vi "Status Tree to JSON.vi"(4 "Status Tree":map{string[], T1}(c390)) -> (7 "JSON":string)   [LabVIEW 2023, in "Volatus.lvlib" / "DebugHTTPController.lvclass"]
uses:
  DebugHTTPController.lvclass
  Module Status.ctl
  Module/State.ctl
  lv-cdm/CDM-Config/Config-JSON/Config-JSON.lvclass
  lv-cdm/CDM-Config/Config Element/Write Variant Value.vi
  DebugHTTPController.lvclass/DebugHTTPController.ctl
  lv-cdm/CDM-Config/Config Manager/Config Manager.lvclass
  lv-cdm/CDM-Config/Config Element/Config Element.lvclass
  Module/Module.lvclass
  Volatus.lvlib
panel:
  out "error out":errorcluster
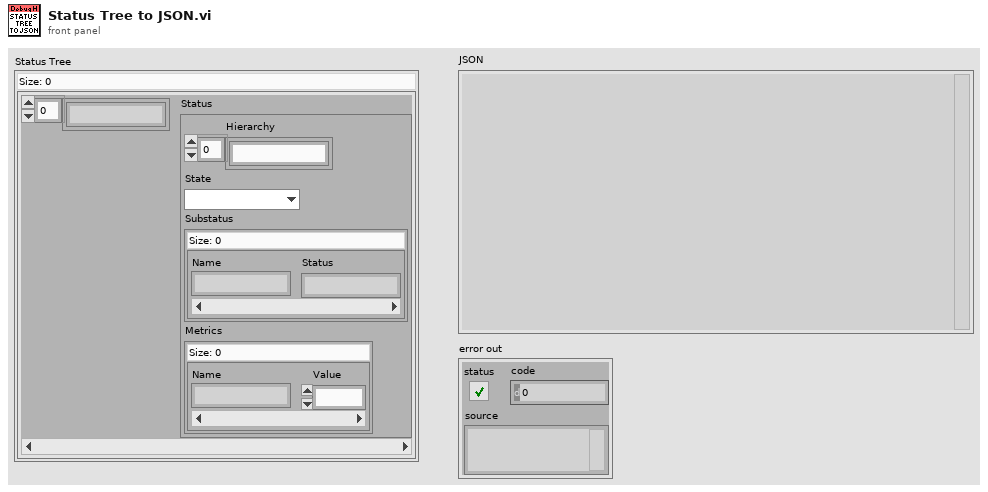
[diagram p1: front panel]
types:
  T1 = typedef "Volatus.lvlib/Module Status.ctl" = cluster{"Hierarchy":string[], "State":T2, "Substatus":map{string, string}, "Metrics":map{string, dbl}}
  T2 = typedef "Volatus.lvlib/Module.lvclass/State.ctl" = enum16{"Unknown", "Launched", "Starting", "Running", "Stopping", "Stopped", "Error - Starting", "Error - Run", "Error - Stopping"}
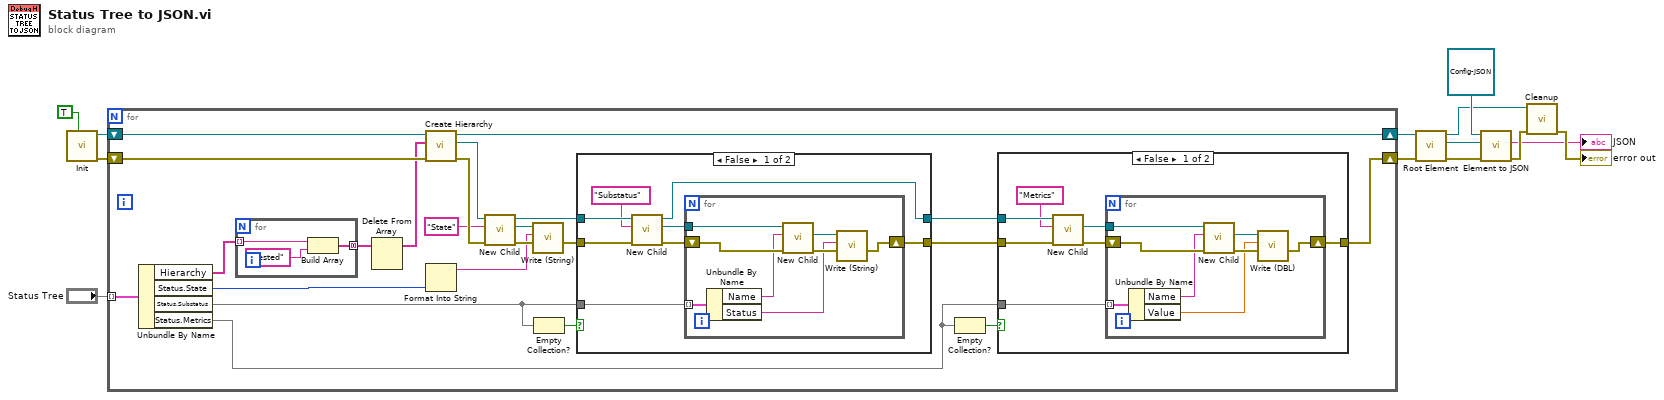
[diagram p0: block diagram]
diagram:
  n1 = call "Init.vi"("Unlock Writes (F)"=TRUE) -> ("error out"=w9:errorcluster, "Config Manager out"=w11:refnum<class "Config Manager.lvclass">)  [unwired: 9 in]
  n2 = for {
    shift-right: [w31] -> w8
    shift-left: w11 -> [w33]
    tunnel: "Status Tree" -> [w34] mode=indexing
    shift-right: [w14] -> w7
    shift-left: w9 -> [w35]
    n3 = Unbundle By Name(w34) -> ("Hierarchy"=w30:string[], "Status.State"=w32:T2, "Status.Substatus"=w22:map{string, string}, "Status.Metrics"=w17:map{string, dbl})
    n4 = for {
      tunnel: w30 -> [w73] mode=indexing
      tunnel: [w71] -> w29 mode=concatenating
      n5 = Build Array(w73, "Nested" ("element")) -> (w71:string[])
    }
    n6 = Delete From Array(array=w29) -> (array with subset deleted=w28:string[])  [unwired: 2 in, 1 out]
    n7 = call "Create Hierarchy.vi"("error in (no error)"=w35, "Hierarchy"=w28, "Config Manager in"=w33) -> ("error out"=w36:errorcluster, "Leaf Element"=w27:refnum<class "Config Element.lvclass">, "Config Manager out"=w31:refnum<class "Config Manager.lvclass">)  [unwired: 6 in]
    n8 = Format Into String(w32) -> (resulting string=w23:string)  [unwired: 3 in, 1 out]
    n9 = call "New Child.vi"("error in (no error)"=w36, "Child Name"="State", "Config Element in"=w27) -> ("error out"=w25:errorcluster, "New Child"=w24:refnum<class "Config Element.lvclass">, "Config Element out"=w20:refnum<class "Config Element.lvclass">)  [unwired: 6 in]
    n10 = call "Write (String).vi"("error in (no error)"=w25, "String Value"=w23, "Config Element in"=w24) -> ("error out"=w19:errorcluster)  [unwired: 7 in, 1 out]
    n11 = Empty Collection?(1:w22) -> (0:w21:bool)
    n12 = case shown="False" w21 {
      tunnel: w22 -> [w55 _]
      tunnel: w20 -> [w59 w69]
      tunnel: w19 -> [w60 w70]
      tunnel: [w54 w70] -> w15
      tunnel: [w53 w69] -> w16
      frame False {
        n13 = call "New Child.vi"("error in (no error)"=w60, "Child Name"="Substatus", "Config Element in"=w59) -> ("error out"=w57:errorcluster, "New Child"=w56:refnum<class "Config Element.lvclass">, "Config Element out"=w53:refnum<class "Config Element.lvclass">)  [unwired: 6 in]
        n14 = for {
          shift-right: [w62] -> w54
          shift-left: w57 -> [w68]
          tunnel: w56 -> [w66]
          tunnel: w55 -> [w67] mode=indexing
          n15 = Unbundle By Name(w67) -> ("Name"=w65:string, "Status"=w61:string)
          n16 = call "New Child.vi"("error in (no error)"=w68, "Child Name"=w65, "Config Element in"=w66) -> ("error out"=w64:errorcluster, "New Child"=w63:refnum<class "Config Element.lvclass">)  [unwired: 6 in, 1 out]
          n17 = call "Write (String).vi"("error in (no error)"=w64, "String Value"=w61, "Config Element in"=w63) -> ("error out"=w62:errorcluster)  [unwired: 7 in, 1 out]
        }
      }
      frame True {
      }
    }
    n18 = Empty Collection?(1:w17) -> (0:w18:bool)
    n19 = case shown="False" w18 {
      tunnel: w17 -> [w38 _]
      tunnel: w16 -> [w42 _]
      tunnel: w15 -> [w43 w52]
      tunnel: [w37 w52] -> w14
      frame False {
        n20 = call "New Child.vi"("error in (no error)"=w43, "Child Name"="Metrics", "Config Element in"=w42) -> ("error out"=w40:errorcluster, "New Child"=w39:refnum<class "Config Element.lvclass">)  [unwired: 6 in, 1 out]
        n21 = for {
          shift-right: [w45] -> w37
          shift-left: w40 -> [w51]
          tunnel: w39 -> [w49]
          tunnel: w38 -> [w50] mode=indexing
          n22 = Unbundle By Name(w50) -> ("Name"=w48:string, "Value"=w44:dbl)
          n23 = call "New Child.vi"("error in (no error)"=w51, "Child Name"=w48, "Config Element in"=w49) -> ("error out"=w47:errorcluster, "New Child"=w46:refnum<class "Config Element.lvclass">)  [unwired: 6 in, 1 out]
          n24 = call "Write (DBL).vi"("error in (no error)"=w47, "DBL Value"=w44, "Config Element in"=w46) -> ("error out"=w45:errorcluster)  [unwired: 7 in, 1 out]
        }
      }
      frame True {
      }
    }
  }
  n25 = call "Root Element.vi"("error in (no error)"=w7, "Config Manager in"=w8) -> ("error out"=w5:errorcluster, "Root Element"=w6:refnum<class "Config Element.lvclass">, "Config Manager out"=w2:refnum<class "Config Manager.lvclass">)  [unwired: 7 in]
  n26 = call "Element to JSON.vi"("error in (no error)"=w5, "Element"=w6, "Config-JSON"=refnum<class "Config-JSON.lvclass"> refnum) -> ("error out"=w13:errorcluster, "JSON"=→"JSON":string)  [unwired: 7 in]
  n27 = call "Cleanup.vi"("error in (no error)"=w13, "Config Manager in"=w2) -> ("error out"=→"error out":errorcluster)  [unwired: 9 in]
